vi "CoordSystem_Convert.vi"(9 "CoordSys To":T1={"Rotation"={"Q_quaternion"={"R"=1.0, "V"=[0.0, 0.0, 0.0]}}}, 10 "CoordSys From":T1={"Rotation"={"Q_quaternion"={"R"=1.0, "V"=[0.0, 0.0, 0.0]}}}, 11 "in Pose3d":T4={"Translation3d"={"X"=0.0, "Y"=0.0, "Z"=0.0}, "Rotation3d"={"Q_quaternion"={"R"=1.0, "V"=[0.0, 0.0, 0.0]}}} {"Translation3d"."Z" format="%14.3f"; "Translation3d"."Y" format="%14.3f"; "Translation3d"."X" format="%14.3f"}) -> (3 "out Converted Pose3d":T4={"Translation3d"={"X"=0.0, "Y"=0.0, "Z"=0.0}, "Rotation3d"={"Q_quaternion"={"R"=1.0, "V"=[0.0, 0.0, 0.0]}}} {"Translation3d"."Z" format="%14.3f"; "Translation3d"."Y" format="%14.3f"; "Translation3d"."X" format="%14.3f"})   [LabVIEW 2019, in "Trajectory_Library.lvlib"]
doc: "Convenience constructors that takes in x and y values directly instead of having to construct a Translation2d.\n\nParameters:\n - X- The x component of the translational component of the pose.\n - Y - The y component of the translational component of the pose.\n - Rotation (Heading) - The rotational component of the pose.\n\nReturns:\n - OUT POSE - Output POSE"
uses:
  ROTATION3D.ctl
  QUATERNION.ctl
  MatBuilder_Create.vi
  Matrix_AssignBlock.vi
  Matrix_Transpose.vi
  Matrix_Ident.vi
  Matrix_IsEqual.vi
  <vilib>/Analysis/baseanly.llb/A x B.vi
  <vilib>/Analysis/baseanly.llb/Real A x B.vi
  Quaternion_New.vi
  Rotation3d_Create_Quaternion.vi
  CoordAxis_New.vi
  MatrixHelper_CoerceSize.vi
  Quaternion_Normalize.vi
  Quaternion_New_Default.vi
  <vilib>/Analysis/7linalg.llb/Create Special Matrix.vi
  <vilib>/Analysis/7linalg.llb/Create Special Real Matrix.vi
  <vilib>/Analysis/Matrix/Numeric/Conversions/Array To Matrix.vi
  <vilib>/Analysis/Matrix/Numeric/Conversions/Array To Matrix - RA.vi
  Trajectory_Library.lvlib
  TRANSLATION3D.ctl
  POSE3D.ctl
  COORDINATE_SYSTEM.ctl
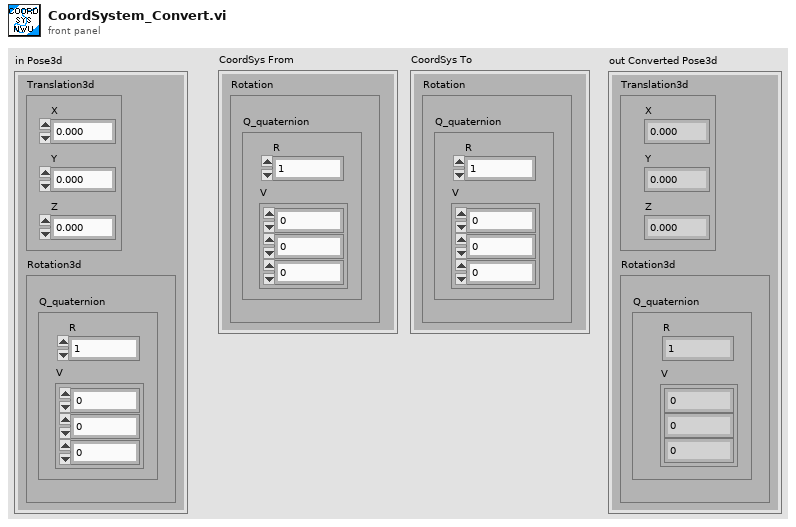
[diagram p1: front panel]
types:
  T1 = typedef "Trajectory_Library.lvlib/COORDINATE_SYSTEM.ctl" = cluster{"Rotation":T2}
  T2 = typedef "Trajectory_Library.lvlib/ROTATION3D.ctl" = cluster{"Q_quaternion":T3}
  T3 = typedef "Trajectory_Library.lvlib/QUATERNION.ctl" = cluster{"R":dbl, "V":dbl[]}
  T4 = typedef "Trajectory_Library.lvlib/POSE3D.ctl" = cluster{"Translation3d":T5, "Rotation3d":T2}
  T5 = typedef "Trajectory_Library.lvlib/TRANSLATION3D.ctl" = cluster{"X":dbl, "Y":dbl, "Z":dbl}
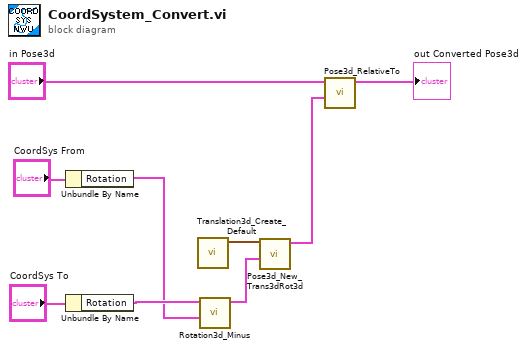
[diagram p0: block diagram]
diagram:
  n1 = Unbundle By Name("CoordSys From") -> ("Rotation"=w6:T2)
  n2 = Unbundle By Name("CoordSys To") -> ("Rotation"=w7:T2)
  n3 = call "Translation3d_Create_Default.vi"() -> ("TRANSLATION3D"=w5:T5)  [unwired: 11 in]
  n4 = call "Rotation3d_Minus.vi"("other Rotation3d"=w6, "in Rotation3d"=w7) -> ("out Rotation3d"=w4:T2)  [unwired: 9 in]
  n5 = call "Pose3d_New_Trans3dRot3d.vi"("Rotation3d"=w4, "Translation3d"=w5) -> ("outPose3d"=w2:T4)  [unwired: 9 in]
  n6 = call "Pose3d_RelativeTo.vi"("other Pose3d"=w2, "in Pose3d"="in Pose3d") -> ("out Pose3d"=→"out Converted Pose3d":T4)  [unwired: 9 in]
